vi "MM9.PG_init.vi"(0 "i ref in":refnum<vi>, 2 "InitObjs":string[](array[string]), 3 "ms timeout (10000)":i32=10000, 5 "error in (no error)":errorcluster) -> (14 "i ref out":refnum<vi>, 16 "InitObjs out":string[](array[string]), 17 "timed out":bool, 19 "error out":errorcluster)   [LabVIEW 2014, in "MM9.lvlib"]
doc: "Initializes the timing pattern generator used."
uses:
  MM9.lvlib
  CS_Core/CAEObj/CAEObj.event definition.ctl
  CS_Core/CSSystem/CoreLib/CoreLib.int 2 byte array.vi
  CS_DigitalIO/PPG_ABC/PPG_ABC.lvlib
  CS_Core/CAEObj/CAEObj.lvlib
  CS_Core/BaseProcess/BaseProcess.lvlib
  CS_Core/CSSystem/CoreLib/CoreLib.lvlib
panel:
  in  "eventDefinition":T1
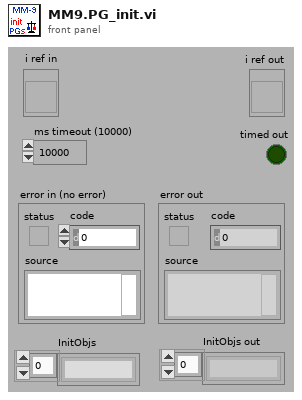
[diagram p1: front panel]
types:
  T1 = typedef "CAEObj.lvlib/CAEObj.event definition.ctl" = cluster{"URL":string, "enable":bool, "ignoreResID":bool}
  T2 = typedef "PPG_ABC.lvlib/PPG_ABC.PG_dataType.ctl" = cluster{"PGDevice":string, "rawPatternData":cluster{"triggerCondition":i32, "timeTable":dbl[], "channelTable":string[]}[]}
  T3 = typedef "CoreDefs.rawDataType.ctl" = i8[]
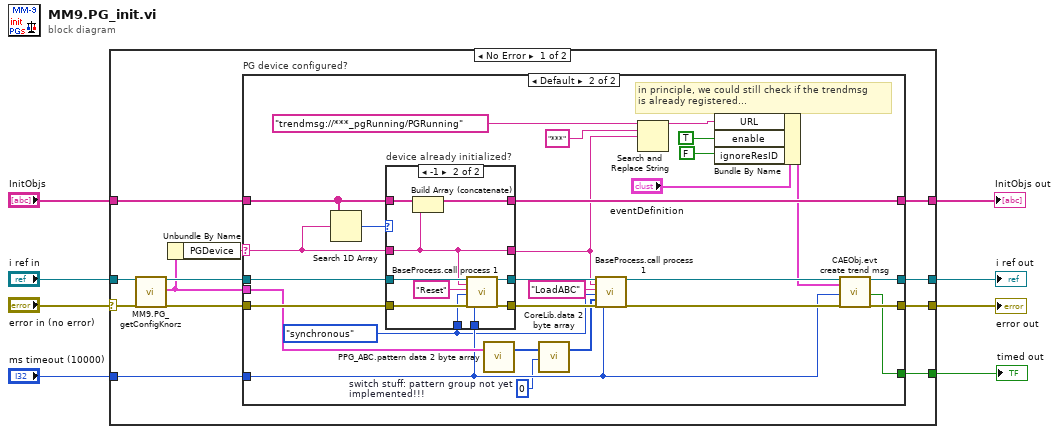
[diagram p0: block diagram]
diagram:
  n1 = case shown="No Error" "error in (no error)" {
    selector: "error in (no error)" -> [w19 w66]
    tunnel: "i ref in" -> [w20 w67]
    tunnel: [w13 w67] -> w7
    tunnel: [w11 w66] -> w6
    tunnel: "InitObjs" -> [w16 w68]
    tunnel: [w12 w68] -> w4
    tunnel: "ms timeout (10000)" -> [w10 _]
    tunnel: [w9 _] -> w1
    frame No Error {
      n2 = call "MM9.PG_getConfigKnorz.vi"("i ref in"=w20, "error in (no error)"=w19) -> ("i ref out"=w17:refnum<vi>, "PGData"=w15:T2, "error out"=w18:errorcluster)  [unwired: 15 in]
      n3 = Unbundle By Name(w15) -> ("PGDevice"=w14:string)
      n4 = case "PG device configured?" shown="Default" w14 {
        selector: w14 -> [_ w49]
        tunnel: w18 -> [w21 w44]
        tunnel: w17 -> [w22 w43]
        tunnel: w16 -> [w23 w50]
        tunnel: w15 -> [_ w42]
        tunnel: [w22 w37] -> w13
        tunnel: [w21 w39] -> w11
        tunnel: [w23 w45] -> w12
        tunnel: w10 -> [_ w27]
        tunnel: [_ w36] -> w9
        frame "" {
        }
        frame Default {
          w26 = enum16{"simple", "synchronous", "asynchronous"}."synchronous" ("CallType")
          w24 = 0  # switch stuff: pattern group not yet implemented!!!
          # "in principle, we could still check if the trendmsg\nis already registered..."
          n5 = Search 1D Array(1D array=w50, element=w49) -> (index of element=w51:i32)  [unwired: 1 in]
          n6 = case "device already initialized?" shown="-1" w51 {
            tunnel: w50 -> [w53 w65]
            tunnel: w49 -> [w52 w58]
            tunnel: w44 -> [w54 w64]
            tunnel: w43 -> [w55 w63]
            tunnel: [w54 w61] -> w47
            tunnel: [w55 w60] -> w48
            tunnel: [w53 w59] -> w45
            tunnel: [w52 w58] -> w33
            tunnel: w27 -> [_ w57]
            tunnel: w26 -> [_ w56]
            frame 0, Default {
            }
            frame -1 {
              n7 = Build Array (concatenate)(w65, w58) -> (w59:string[])
              n8 = call "BaseProcess.call process 1.vi"("i ref in"=w63, "Object"=w58, "Selector"="Reset", "CallType"=w56, "error in (no error)"=w64, "timeout (ms)"=w57) -> ("i ref out"=w60:refnum<vi>, "error out"=w61:errorcluster)  [unwired: 11 in, 1 out]
            }
          }
          n9 = call "PPG_ABC.pattern data 2 byte array.vi"("PGData"=w42) -> ("byteArray out"=w41:T3)  [unwired: 18 in]
          n10 = call-poly "CoreLib.data 2 byte array.vi"("byteArray"=w41, "i32"=w24) -> ("byteArray out"=w25:T3)  [unwired: 17 in]
          n11 = call "BaseProcess.call process 1.vi"("i ref in"=w48, "Object"=w33, "Selector"="LoadABC", "CallType"=w26, "Data"=w25, "error in (no error)"=w47, "timeout (ms)"=w27) -> ("i ref out"=w38:refnum<vi>, "error out"=w40:errorcluster)  [unwired: 10 in, 1 out]
          n12 = Search and Replace String(input string="trendmsg://***_pgRunning/PGRunning", search string="***", replace string=w33) -> (result string=w31:string)  [unwired: 5 in, 3 out]
          n13 = Bundle By Name(cluster="eventDefinition", "URL"=w31, "enable"=TRUE, "ignoreResID"=FALSE) -> (w29:T1)
          n14 = call "CAEObj.evt create trend msg.vi"("i ref in"=w38, "event definition"=w29, "ms timeout (10000)"=w27, "error in (no error)"=w40) -> ("i ref out"=w37:refnum<vi>, "timed out"=w36:bool, "error out"=w39:errorcluster)  [unwired: 12 in, 1 out]
        }
      }
    }
    frame Error {
    }
  }
  "error out" <- w6
  "i ref out" <- w7
  "timed out" <- w1
  "InitObjs out" <- w4
